vi "Read Offline Data.vi"() -> ()   [LabVIEW 2014, in "Aquisicao de Dados.lvlib"]
uses:
  Aquisicao de Dados.lvlib
  <vilib>/Waveform/WDTOps.llb/WDT Number of Waveform Samples DBL.vi
  <vilib>/express/express analysis/Spectral/Block/exnSpectralBlock spectral measurements peak poly.vi
  <vilib>/express/express analysis/Spectral/Block/exnSpectralBlock spectral measurements peak WFM.vi
  <vilib>/Waveform/WDTOps.llb/WDT Get Waveform Subset DBL.vi
  <vilib>/Waveform/WDTOps.llb/WDT Waveform Duration DBL.vi
  <vilib>/express/express analysis/Spectral/XNode/ExpressSpectralMeasurementsBlockNode.xnode
panel:
  out "Frequência":dbl
  out "Periodo de\namostragem(Td)":dbl
  out "Taxa de \namostragem(Fs)":dbl
  out "Número total \nde amostras":i32
  out "Menor amplitude":dbl format="%0.2f"
  out "Maior amplitude":dbl format="%0.2f"
  out "RMS":dbl
  out "Valor PP":dbl
  in  "Stop Button":bool
  out "Sinal  Completo":waveform(dbl)(graph)
  out "Espectro Completo":cluster{"f0":dbl, "df":dbl, "magnitude":dbl[]}(graph)
  out "Início":dbl format="%0.2f"
  out "duração":dbl=1.0 format="%0.2f"
  out "Janela no tempo":waveform(dbl)(graph)
  in  "Duração":dbl(slide) scale=0.0..7.677637500000021
  in  "Início":dbl(slide) scale=0.0..9.8431249999999
  out "Fd":dbl
  out "Td":dbl format="%0.2f"
  out "n° de \namostras\n(janela)":i32
  out "Janela espetral":cluster{"f0":dbl, "df":dbl, "magnitude":dbl[]}(graph)
  out "Error Out":errorcluster
  in  "Error In":errorcluster
  # "PSI3214"
  # "Laboratório de Instrumentação Elétrica"
  # "Turma 3"
  # "Professores: Bete e Sandro"
  # "Joaquim Afonso Bacellar Batista de Siqueira\nLeonardo Isao Komura \nVanderson da Silva dos Santos"
  # "Alunos:"
  # "Dados ADC"
  # "Dados Sinal"
  # "Dados Janelamento"
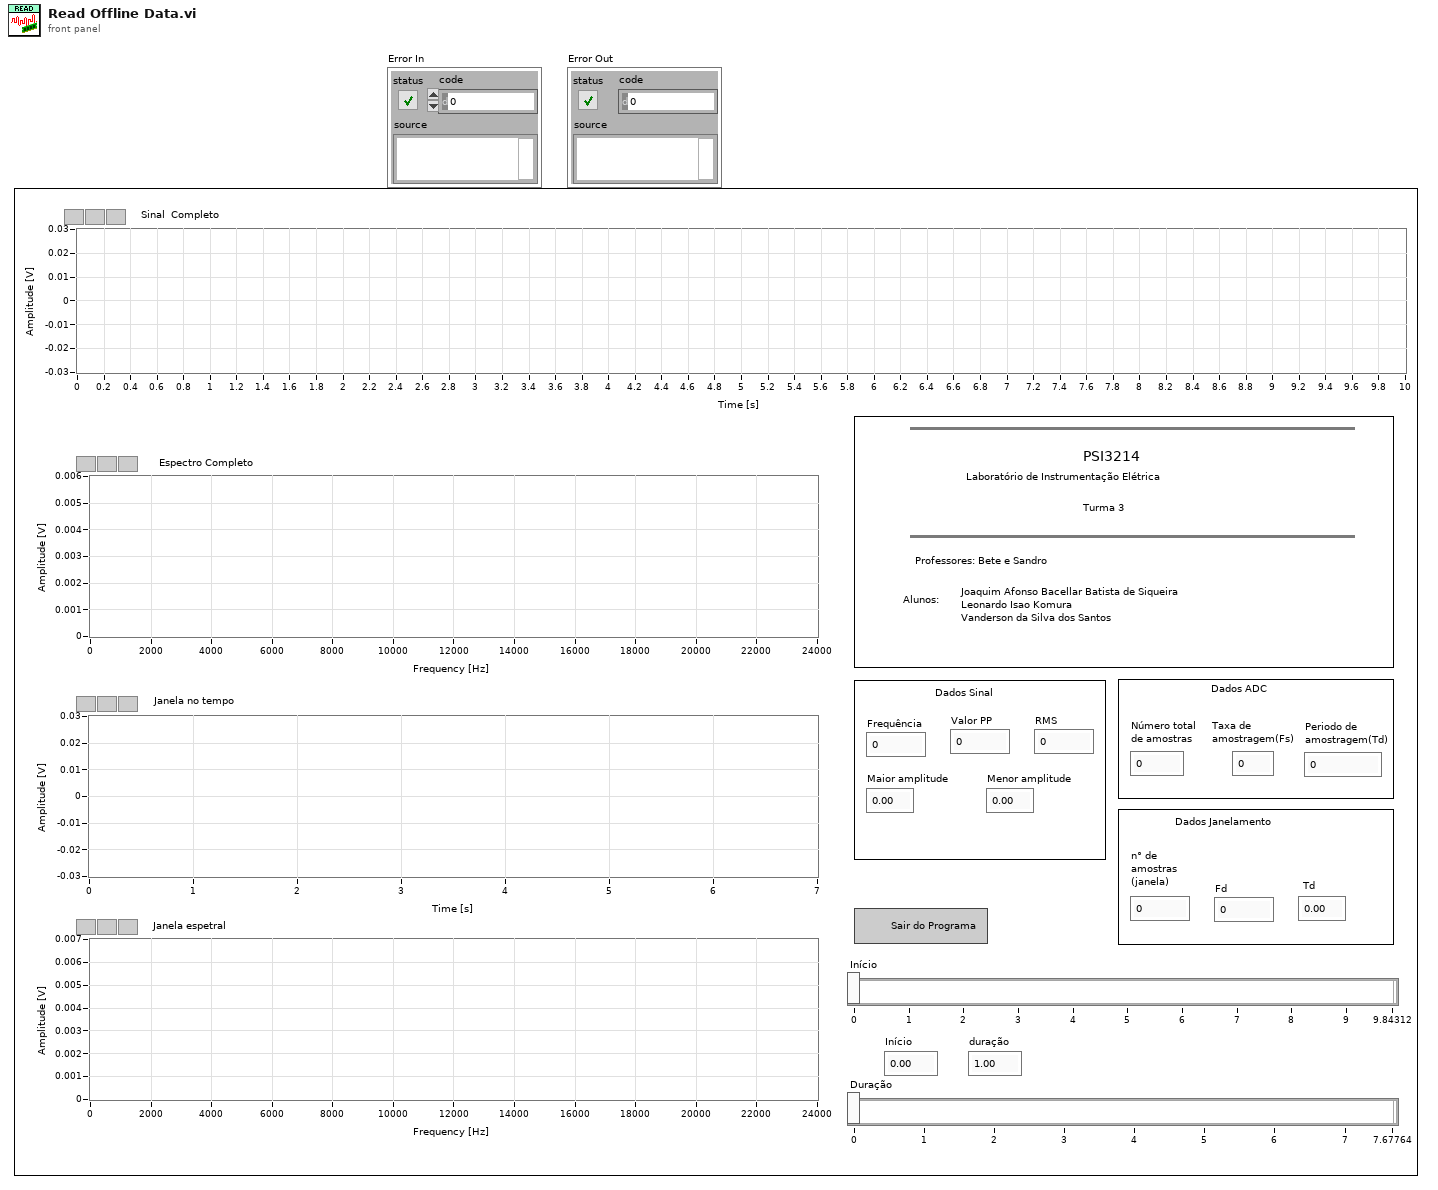
[diagram p1: front panel]
types:
  T1 = enum32{".WAV File", "LTSpice Simulation", "Microphone", "MultiSim Simulation", "Serial Port"}
  T2 = typedef "Aquisicao de Dados.lvlib/_ACC_DATA_ Config DAta State.ctl" = cluster{"_RAW_ Traces":cluster{"Trace Name":string, "Trace Type":string, "Trace Raw Data":dbl[], "Trace Waveform":waveform(dbl)}[], "_WAV_ Traces":waveform(dbl)[], "_MIC_ Config":cluster{"task ID":T3, "Data Chunk Size":i32, "Num Channels":i32, "Resolution":i32, "Sampling Frequency":dbl, "device ID":u32, "Num Chunks":i32}, "_LVM_ Traces":cluster{"Trace Name":string, "Trace Type":string, "Trace Raw Data":dbl[], "Trace Waveform":waveform(dbl)}[]}
  T3 = typedef "Sound Input Task ID.ctl" = u32
  T4 = cluster{"averaging mode":u16, "weighting mode":u16, "number of averages":u32}
  T5 = cluster{"dB On (F)":bool, "unwrap phase (F)":bool, "convert to degree (F)":bool}
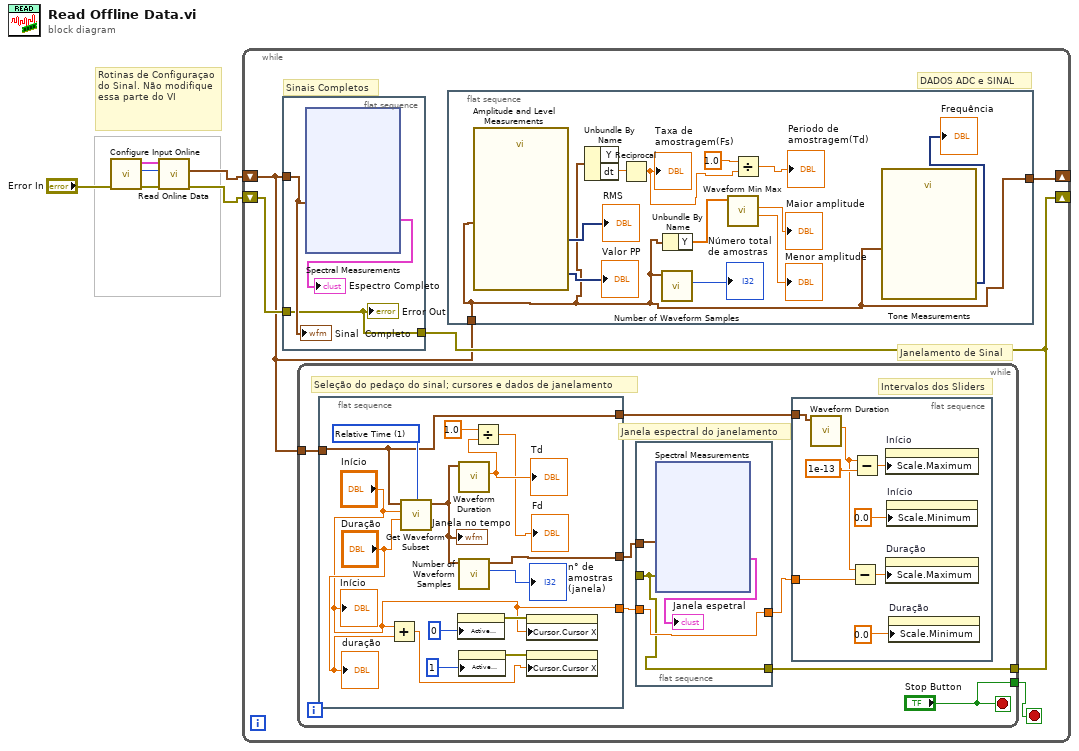
[diagram p0: block diagram]
diagram:
  # "Rotinas de Configuraçao do Sinal. Não modifique essa parte do VI"
  n1 = call "Configure Input Online.vi"("Error In"="Error In") -> ("Error Out"=w3:errorcluster, "Metodo de Entrada"=w5:T1, "Config Out"=w6:T2)  [unwired: 8 in]
  n2 = call "Read Online Data.vi"("Error In"=w3, "Metodo de Entrada"=w5, "Config Out"=w6) -> ("Error Out"=w1:errorcluster, "Channel 0"=w2:waveform(dbl))  [unwired: 6 in, 1 out]
  n3 = while {
    shift-right: [w8] -> _
    shift-left: w2 -> [w7]
    shift-right: [w10] -> _
    shift-left: w1 -> [w11]
    stop <- w9 stop-if-true
    # "Janelamento de Sinal"
    # "DADOS ADC e SINAL"
    # "Sinais Completos"
    n4 = flat-sequence {
      tunnel: w7 -> [w25]
      tunnel: w11 -> [w24]
      tunnel: [w24] -> w10
      frame #0 {
        n5 = xnode "Spectral Measurements"("Signals"=w25) -> ("FFT - (Peak)"=→"Espectro Completo":cluster{"f0":dbl, "df":dbl, "magnitude":dbl[]})  [unwired: 1 in, 2 out]
        "Error Out" <- w24
        "Sinal  Completo" <- w25
      }
    }
    n6 = while {
      tunnel: w7 -> [w40]
      tunnel: w10 -> [w38]
      tunnel: ["Stop Button"] -> w9
      stop <- "Stop Button" stop-if-true
      # "Janela espectral do janelamento"
      # "Seleção do pedaço do sinal; cursores e dados de janelamento"
      # "Intervalos dos Sliders"
      n7 = flat-sequence {
        tunnel: w40 -> [w58]
        tunnel: [w60] -> w43
        tunnel: ["Início"] -> w42
        tunnel: [w58] -> w39
        frame #0 {
          w72 = u16 1 items=["Samples", "Relative Time"] ("start/duration format")
          n8 = Add(x="Início", y="Duração") -> (x+y=w66:dbl)
          n9 = call-poly <vilib>:"Get Waveform Subset.vi"("start/duration format"=w72, "duration"="Duração", "start samples/time"="Início", "waveform in"=w58) -> ("waveform out"=w64:waveform(dbl))  [unwired: 2 in, 3 out]
          "Janela no tempo" <- w64
          n10 = property on="Sinal  Completo" class="WFGraph (strict)"("Active Cursor"=u32 0) -> (error out=w68:errorcluster)  [unwired: 2 in, 1 out]
          n11 = call-poly <vilib>:"Waveform Duration.vi"("waveform in"=w64) -> ("duration"=w63:dbl)  [unwired: 8 in, 2 out]
          "Td" <- w63
          n12 = call-poly <vilib>:"Number of Waveform Samples.vi"("waveform in"=w64) -> ("number of samples"=→"n° de \namostras\n(janela)":i32, "waveform out"=w60:waveform(dbl))  [unwired: 8 in, 1 out]
          n13 = property on="Sinal  Completo" class="WFGraph (strict)"("Active Cursor"=u32 1) -> (error out=w70:errorcluster)  [unwired: 2 in, 1 out]
          n14 = Divide(x=1.0, y=w63) -> (x/y=→"Fd":dbl)
          n15 = property on="Sinal  Completo" class="WFGraph (strict)"(error in=w68, "Cursor.Cursor X"="Início") -> ()  [unwired: 1 in, 2 out]
          n16 = property on="Sinal  Completo" class="WFGraph (strict)"(error in=w70, "Cursor.Cursor X"=w66) -> ()  [unwired: 1 in, 2 out]
          "duração" <- "Duração"
          "Início" <- "Início"
        }
      }
      n17 = flat-sequence {
        tunnel: w43 -> [w47]
        tunnel: [w44] -> _
        tunnel: w42 -> [w45]
        tunnel: [w45] -> w41
        tunnel: w38 -> [w44]
        frame #0 {
          n18 = xnode "Spectral Measurements"("Signals"=w47, "error in (no error)"=w44) -> ("FFT - (Peak)"=→"Janela espetral":cluster{"f0":dbl, "df":dbl, "magnitude":dbl[]})  [unwired: 2 out]
        }
      }
      n19 = flat-sequence {
        tunnel: w41 -> [w74]
        tunnel: w39 -> [w73]
        frame #0 {
          n20 = call-poly <vilib>:"Waveform Duration.vi"("waveform in"=w73) -> ("duration"=w76:dbl)  [unwired: 8 in, 2 out]
          n21 = Subtract(x=w76, y=w74) -> (x-y=w77:dbl)
          n22 = Subtract(x=w76, y=1e-13) -> (x-y=w80:dbl)
          n23 = property on="Início" class="Slide (strict)"("Scale.Maximum"=w80) -> ()  [unwired: 2 in, 2 out]
          n24 = property on="Duração" class="Slide (strict)"("Scale.Maximum"=w77) -> ()  [unwired: 2 in, 2 out]
          n25 = property on="Início" class="Slide (strict)"("Scale.Minimum"=0.0 ("Scale.Range:Minimum")) -> ()  [unwired: 2 in, 2 out]
          n26 = property on="Duração" class="Slide (strict)"("Scale.Minimum"=0.0 ("Scale.Range:Minimum")) -> ()  [unwired: 2 in, 2 out]
        }
      }
    }
    n27 = flat-sequence {
      tunnel: [w12] -> w8
      tunnel: w7 -> [w12]
      frame #0 {
        n28 = call "Amplitude and Level Measurements"("Signals"=w12) -> ("RMS"=→"RMS":dynamicdata, "Peak to Peak"=→"Valor PP":dynamicdata)  [unwired: 12 in, 1 out]
        n29 = Unbundle By Name ("Get Waveform Components")(w12) -> ("dt"=w22:dbl)  [unwired: 1 out]
        n30 = Reciprocal(x=w22) -> (1/x=w15:dbl)
        "Taxa de \namostragem(Fs)" <- w15
        n31 = call-poly <vilib>:"Number of Waveform Samples.vi"("waveform in"=w12) -> ("number of samples"=→"Número total \nde amostras":i32)  [unwired: 8 in, 2 out]
        n32 = Unbundle By Name(w12) -> ("Y"=w19:dbl[])
        n33 = call <vilib>:"Waveform Min Max.vi"("waveform in"=w19) -> ("Y min"=→"Menor amplitude":dbl, "Y max"=→"Maior amplitude":dbl)  [unwired: 5 in, 4 out]
        n34 = Divide(x=1.0, y=w15) -> (x/y=→"Periodo de\namostragem(Td)":dbl)
        n35 = call "Tone Measurements"("Signals"=w12) -> ("Frequency"=→"Frequência":dynamicdata)  [unwired: 8 in, 2 out]
      }
    }
  }
